vi "runscenario expand OR query value.vi"(11 "Value String":string) -> (1 "Items?":bool, 2 "Value OR String":string, 3 "Value Item Array":string[](array[string]))   [LabVIEW 2011]
panel:
  out "Ranges Array":string[](array[string])
  # "Things to test if you change this...\nTest Empty String = No Elements\nTest two or more spaces   =  No Elements\n,,,,= [] (No Elements)\n, , , = [] (No Elements)\n1,2,4-7 = [1,2,4,5,6,7]\nA4-7 =  [A4-7]\nA 4-7= [A 4- 7]\nA 4   -    A 7 = [A4,A5,A6,A7]\nA-10-A-11 = [A-10, A-11]\nS/N 3 = [S/N 3]\nA-10 = [A-10]\na-r10 = [a-r10]\nA3-4 = [A3-4]\nA3-A4 = [A3,A4]\n-A3 = [-A3]\n--A3 = [--A3]\n-A3-1 = [-A3-1]\n-A3-3 = [-A3-3]\n-A3-4 = [-A3,-A4]\n-A3-4- = [-A3-4-]\n-A3-4-5 = [-A3-4, -A3-5]\n-A3-4-4 = [-A3-4-4]\nPre - fix 4-   Pre - fix 7 = [Pre  - fix  4,Pre  - fix  5,Pre  - fix  6,Pre  - fix  7]\n* = [] (No Elements)\n? = [] (No Elements)\n$SSN$ 0000000000000001-3 =[$SSN$  0000000000000001,$SSN$  0000000000000002,$SSN$  0000000000000003]\n0005-0008 = [0005,0006, 0007, 0008]\n009-012 = [009, 010,011,012]\na-1-28-a-1-32 = [a-1-28,a-1-29,a-1-30, a-1-31, a-1-32]"
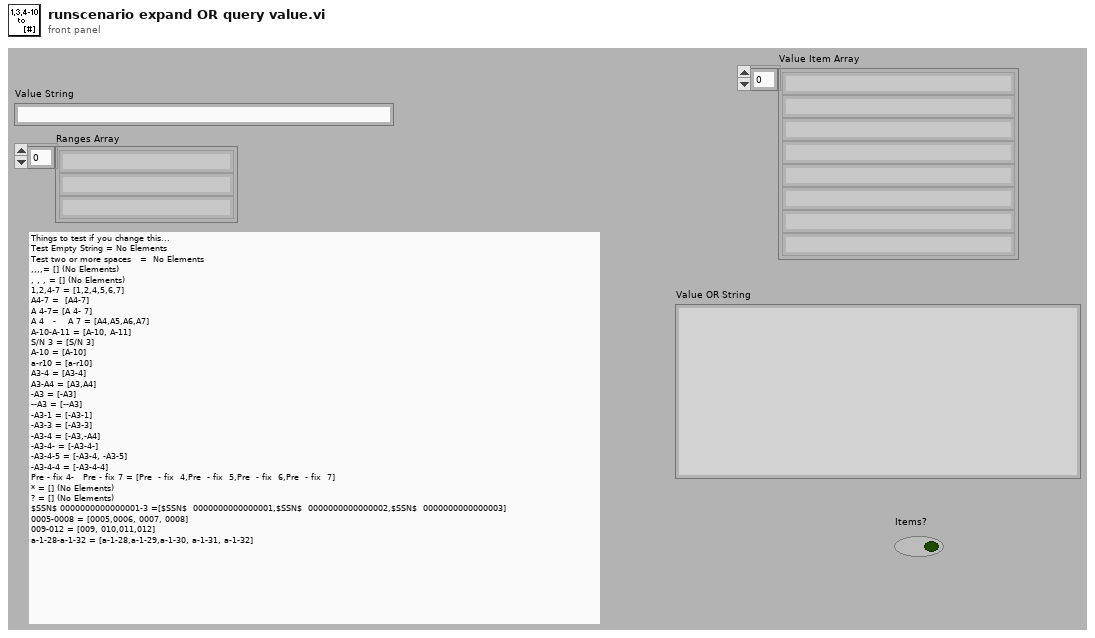
[diagram p1: front panel]
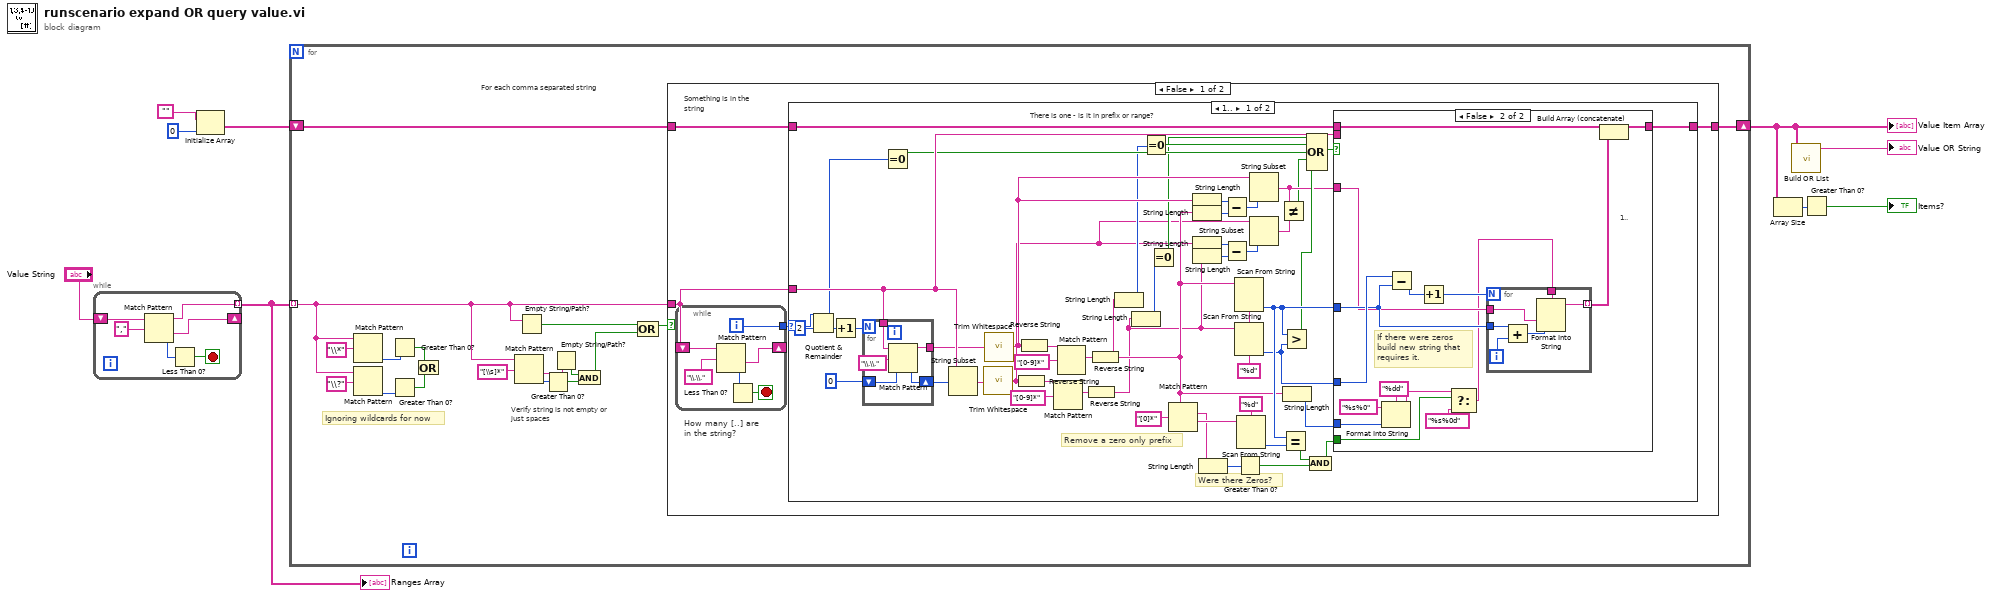
[diagram p0: block diagram]
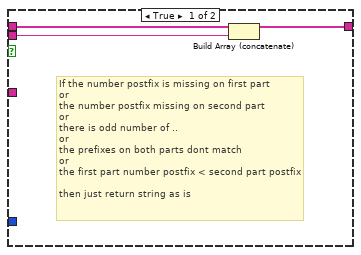
[diagram p2: hidden frame]
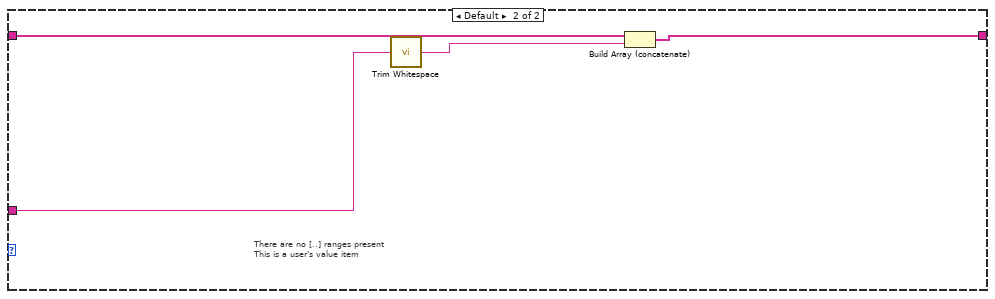
[diagram p3: hidden frame]
diagram:
  n1 = while {
    shift-right: [w10] -> _
    shift-left: "Value String" -> [w15]
    tunnel: [w13] -> w9 mode=indexing
    stop <- w12 stop-if-true
    n2 = Match Pattern(string=w15, regular expression=",") -> (before substring=w13:string, after substring=w10:string, offset past match=w11:i32)  [unwired: 2 out]
    n3 = Less Than 0?(x=w11) -> (x < 0?=w12:bool)
  }
  "Ranges Array" <- w9
  n4 = Initialize Array("", 0) -> (w5:string[])
  n5 = for {
    tunnel: w9 -> [w24] mode=indexing
    shift-right: [w31] -> w2
    shift-left: w5 -> [w32]
    # "Ignoring wildcards for now"
    # "Verify string is not empty or\njust spaces"
    # "For each comma separated string"
    n6 = Match Pattern(string=w24, regular expression="\\*" ("format string")) -> (offset past match=w26:i32)  [unwired: 4 out]
    n7 = Match Pattern(string=w24, regular expression="\\?" ("format string")) -> (offset past match=w25:i32)  [unwired: 4 out]
    n8 = Greater Than 0?(x=w26) -> (x > 0?=w28:bool)
    n9 = Greater Than 0?(x=w25) -> (x > 0?=w29:bool)
    n10 = Or(x=w28, y=w29) -> ()  [unwired: 1 out]
    n11 = Match Pattern(string=w24, regular expression="[\\s]*" ("format string")) -> (after substring=w19:string, offset past match=w20:i32)  [unwired: 3 out]
    n12 = Empty String/Path?(string/path=w24) -> (empty?=w22:bool)
    n13 = Greater Than 0?(x=w20) -> (x > 0?=w17:bool)
    n14 = Empty String/Path?(string/path=w19) -> (empty?=w18:bool)
    n15 = And(x=w18, y=w17) -> (x .and. y?=w16:bool)
    n16 = Compound Arithmetic op=OR(w22, w16) -> (w21:bool)
    n17 = case shown="False" w21 {
      tunnel: w24 -> [w34 _]
      tunnel: w32 -> [w36 w127]
      tunnel: [w35 w127] -> w31
      frame False {
        # "How many [..] are\nin the string?"
        # "Something is in the \nstring"
        n18 = while {
          tunnel: [w39] -> w33
          shift-right: [w38] -> _
          shift-left: w34 -> [w37]
          i -> [w39]
          stop <- w40 stop-if-true
          n19 = Match Pattern(string=w37, regular expression="\\.\\.") -> (after substring=w38:string, offset past match=w41:i32)  [unwired: 3 out]
          n20 = Less Than 0?(x=w41) -> (x < 0?=w40:bool)
        }
        n21 = case shown="1.." w33 {
          selector: w33 -> [w76 _]
          tunnel: w34 -> [w74 w124]
          tunnel: w36 -> [w93 w126]
          tunnel: [w92 w125] -> w35
          frame 1.. {
            w65 = "%d" ("format string")
            # "Were there Zeros?"
            # "Remove a zero only prefix"
            # "There is one - is it in prefix or range?"
            n22 = Quotient & Remainder(x=w76, y=2) -> (x-y*floor(x/y)=w57:i32, floor(x/y)=w78:i32)
            n23 = Increment(x=w78) -> (x+1=w80:i32)
            n24 = for {
              N: w80 -> [_]
              shift-right: [w97] -> w75
              shift-left: 0 ("y") -> [w98]
              tunnel: [w95] -> w73
              tunnel: w74 -> [w94]
              n25 = Match Pattern(string=w94, regular expression="\\.\\.", offset (0)=w98) -> (before substring=w95:string, offset past match=w97:i32)  [unwired: 2 out]
            }
            n26 = Equal To 0?(x=w57) -> (x = 0?=w56:bool)
            n27 = String Subset(string=w74, offset (0)=w75) -> (substring=w72:string)  [unwired: 1 out]
            n28 = call <vilib>:"Trim Whitespace.vi"("string"=w72) -> ("trimmed string"=w43:string)  [unwired: 1 in]
            n29 = call <vilib>:"Trim Whitespace.vi"("string"=w73) -> ("trimmed string"=w63:string)  [unwired: 1 in]
            n30 = Reverse String(1:w43) -> (0:w67:string)
            n31 = Reverse String(1:w63) -> (0:w70:string)
            n32 = Match Pattern(string=w67, regular expression="[0-9]*" ("format string")) -> (match substring=w66:string)  [unwired: 4 out]
            n33 = Match Pattern(string=w70, regular expression="[0-9]*" ("format string")) -> (match substring=w71:string)  [unwired: 4 out]
            n34 = Reverse String(1:w66) -> (0:w44:string)
            n35 = Reverse String(1:w71) -> (0:w55:string)
            n36 = String Length(string=w55) -> (length=w54:i32)
            n37 = String Length(string=w44) -> (length=w52:i32)
            n38 = Equal To 0?(x=w54) -> (x = 0?=w53:bool)
            n39 = Equal To 0?(x=w52) -> (x = 0?=w51:bool)
            n40 = Match Pattern(string=w55, regular expression="[0]*" ("format string")) -> (match substring=w82:string, after substring=w89:string)  [unwired: 3 out]
            n41 = String Length(string=w63) -> (length=w62:i32)
            n42 = String Length(string=w55) -> (length=w61:i32)
            n43 = String Length(string=w43) -> (length=w48:i32)
            n44 = String Length(string=w44) -> (length=w49:i32)
            n45 = String Length(string=w82) -> (length=w81:i32)
            n46 = Subtract(x=w62, y=w61) -> (x-y=w60:i32)
            n47 = Subtract(x=w48, y=w49) -> (x-y=w50:i32)
            n48 = Scan From String(format string=w65, input string=w55) -> (output 1=w87:i32)  [unwired: 2 in, 4 out]
            n49 = Scan From String(format string=w65, input string=w44) -> (output 1=w64:i32)  [unwired: 2 in, 4 out]
            n50 = Greater Than 0?(x=w81) -> (x > 0?=w83:bool)
            n51 = Scan From String(format string="%d", input string=w89) -> (output 1=w88:i32)  [unwired: 2 in, 4 out]
            n52 = String Subset(string=w63, length (rest)=w60) -> (substring=w46:string)  [unwired: 1 out]
            n53 = String Subset(string=w43, length (rest)=w50) -> (substring=w47:string)  [unwired: 1 out]
            n54 = Not Equal?(x=w46, y=w47) -> (x != y?=w45:bool)
            n55 = Equal?(x=w87, y=w88) -> (x = y?=w85:bool)
            n56 = Greater?(x=w87, y=w64) -> (0:w59:bool)
            n57 = String Length(string=w55) -> (length=w86:i32)
            n58 = Compound Arithmetic op=OR(w51, w53, w56, w45, w59) -> (w58:bool)
            n59 = And(x=w85, y=w83) -> (x .and. y?=w84:bool)
            n60 = case shown="False" w58 {
              tunnel: w64 -> [_ w116]
              tunnel: w87 -> [_ w114]
              tunnel: w93 -> [w101 w112]
              tunnel: [w100 w111] -> w92
              tunnel: w74 -> [w99 _]
              tunnel: w86 -> [_ w108]
              tunnel: w84 -> [_ w105]
              tunnel: w46 -> [_ w103]
              frame True {
                # "If the number postfix is missing on first part\nor\nthe number postfix missing on second part \nor\nthere is odd number of ..\nor\nthe prefixes on both parts dont match\nor\nthe first part number postfix < second part postfix\n\nthen just return string as is"
                n61 = Build Array (concatenate)(w101, w99) -> (w100:string[])
              }
              frame False {
                # "If there were zeros\nbuild new string that \nrequires it."
                # "1.."
                n62 = Format Into String(format string="%dd", initial string="%s%0" ("format string"), w108) -> (resulting string=w104:string)  [unwired: 1 in, 1 out]
                n63 = Subtract(x=w116, y=w114) -> (x-y=w115:i32)
                n64 = Increment(x=w115) -> (x+1=w110:i32)
                n65 = Select(t=w104, s=w105, f="%s%0d" ("format string")) -> (s? t:f=w102:string)
                n66 = for {
                  N: w110 -> [_]
                  tunnel: w114 -> [w122]
                  tunnel: w103 -> [w119]
                  tunnel: [w118] -> w113 mode=indexing
                  tunnel: w102 -> [w117]
                  i -> [w121]
                  n67 = Add(x=w122, y=w121) -> (x+y=w120:i32)
                  n68 = Format Into String(format string=w117, w119, w120) -> (resulting string=w118:string)  [unwired: 2 in, 1 out]
                }
                n69 = Build Array (concatenate)(w112, w113) -> (w111:string[])
              }
            }
          }
          frame Default {
            # "There are no [..] ranges present\nThis is a user's value item"
            n70 = call <vilib>:"Trim Whitespace.vi"("string"=w124) -> ("trimmed string"=w123:string)  [unwired: 1 in]
            n71 = Build Array (concatenate)(w126, w123) -> (w125:string[])
          }
        }
      }
      frame True {
        # "Don't process an empty string or a string composes of spaces."
      }
    }
  }
  "Value Item Array" <- w2
  n72 = Array Size(array=w2) -> (size(s)=w4:i32)
  n73 = call "Build OR List.vi"("String Array"=w2) -> ("OR String"=→"Value OR String":string)  [unwired: 10 out]
  n74 = Greater Than 0?(x=w4) -> (x > 0?=→"Items?":bool)
